vi "Read FAN3.vi"(8 "error in (no error)":errorcluster, 11 "ParameterConf in":refnum<class "ParameterConf.lvclass">) -> (0 "error out":errorcluster, 1 "Queue Process.Serial Data Gcode":refnum<queue>, 2 "FAN3":dbl min=0.0 max=255.0 step=5.0, 3 "ParameterConf out":refnum<class "ParameterConf.lvclass">)   [LabVIEW 2017, in "LibraryGcode.lvlib" / "ParameterConf.lvclass"]
uses:
  ParameterConf.lvclass
  ParameterConf.lvclass/ParameterConf.ctl
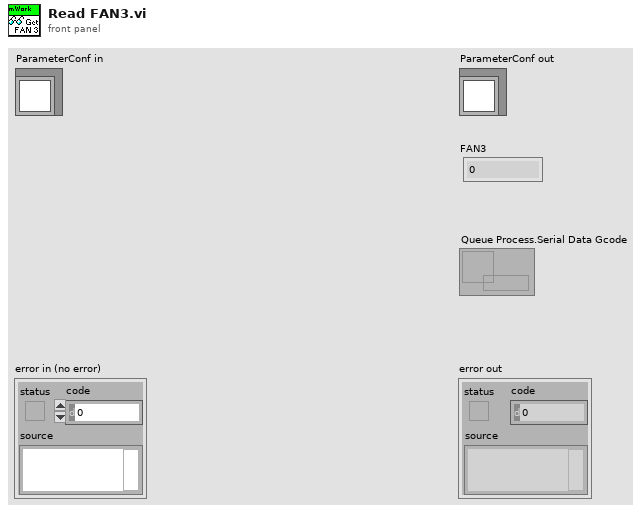
[diagram p1: front panel]
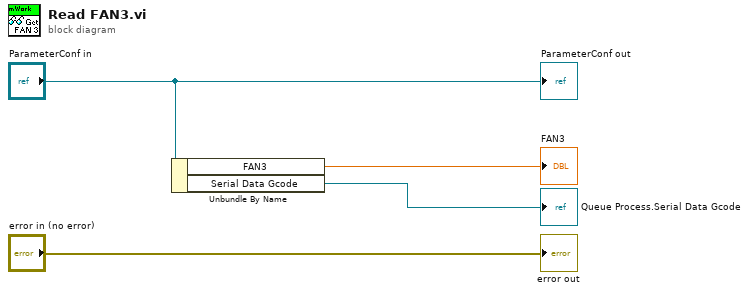
[diagram p0: block diagram]
diagram:
  n1 = Unbundle By Name("ParameterConf in") -> ("FAN3"=→"FAN3":dbl, "Serial Data Gcode"=→"Queue Process.Serial Data Gcode":refnum<queue>)
  "error out" <- "error in (no error)"
  "ParameterConf out" <- "ParameterConf in"
